vi "setColors.vi"(8 "error in (no error)":errorcluster, 10 "Colors":T1, 11 "Theme in":refnum<class "Theme.lvclass">) -> (0 "error out":errorcluster, 3 "Theme out":refnum<class "Theme.lvclass">)   [LabVIEW 2017, in "Theme.lvlib" / "Theme.lvclass"]
uses:
  Theme.lvclass
  Theme.Colors/Colors.ctl
  Theme.Colors/Theme.Colors.lvclass
  Theme.Colors/Theme.Colors.lvclass/Theme.Colors.ctl
  Theme.lvclass/Theme.ctl
  Theme.Colors/setContainer.vi
  Theme.Colors/setMain.vi
  Theme.Colors/setText.vi
  Theme.Font/Theme.Font.lvclass
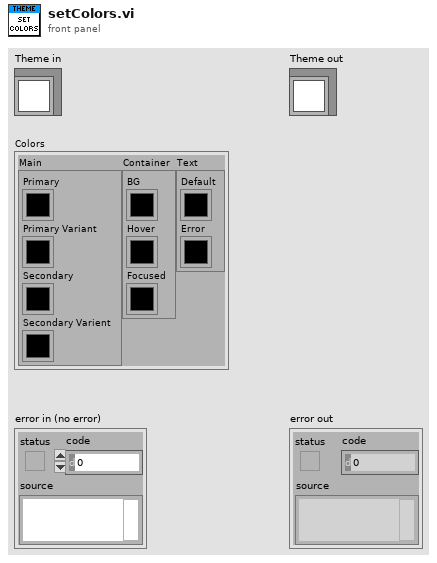
[diagram p1: front panel]
types:
  T1 = typedef "Theme.lvlib/Theme.Colors.lvclass/Colors.ctl" = cluster{"Main":cluster{"Primary":u32, "Primary Variant":u32, "Secondary":u32, "Secondary Varient":u32}, "Container":cluster{"BG":u32, "Hover":u32, "Focused":u32}, "Text":cluster{"Default":u32, "Error":u32}}
  T2 = typedef "Theme.lvlib/Theme.lvclass/Private Data.ctl" = cluster{"Colors":refnum<class "Theme.Colors.lvclass">, "Font":refnum<class "Theme.Font.lvclass">}
  T3 = cluster{"Primary":u32, "Primary Variant":u32, "Secondary":u32, "Secondary Varient":u32}
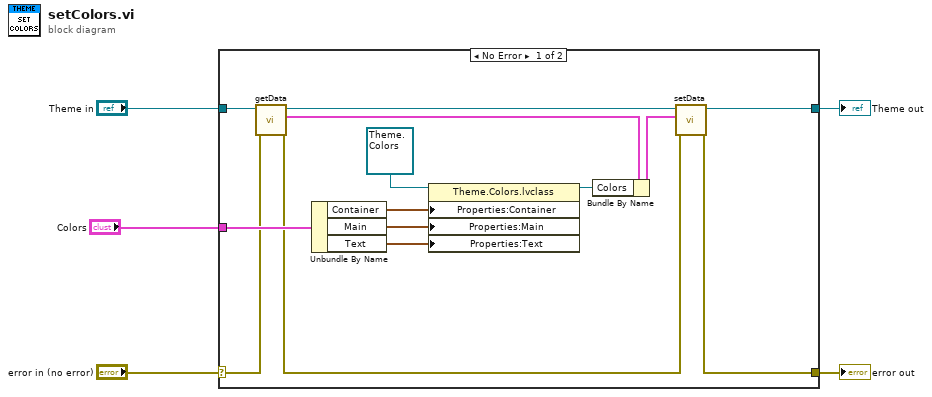
[diagram p0: block diagram]
diagram:
  n1 = case shown="No Error" "error in (no error)" {
    selector: "error in (no error)" -> [w8 w21]
    tunnel: [w6 w21] -> w4
    tunnel: [w18 w20] -> w2
    tunnel: "Theme in" -> [w17 w20]
    tunnel: "Colors" -> [w12 _]
    frame No Error {
      n2 = call "getData.vi"("error in (no error)"=w8, "Theme in"=w17) -> ("error out"=w7:errorcluster, "Theme"=w16:T2, "Theme out"=w19:refnum<class "Theme.lvclass">)  [unwired: 7 in]
      n3 = Unbundle By Name(w12) -> ("Container"=w11:cluster{"BG":u32, "Hover":u32, "Focused":u32}, "Main"=w10:T3, "Text"=w9:cluster{"Default":u32, "Error":u32})
      n4 = property class="Theme.Colors.lvclass"(reference=refnum<class "Theme.Colors.lvclass"> refnum ("Theme.lvlib:Theme.Colors.lvclass"), "Properties:Container"=w11, "Properties:Main"=w10, "Properties:Text"=w9) -> (reference out=w13:refnum<class "Theme.Colors.lvclass">)  [unwired: 1 in, 1 out]
      n5 = Bundle By Name(cluster=w16, "Colors"=w13) -> (w15:T2)
      n6 = call "setData.vi"("error in (no error)"=w7, "Theme"=w15, "Theme in"=w19) -> ("error out"=w6:errorcluster, "Theme out"=w18:refnum<class "Theme.lvclass">)  [unwired: 7 in]
    }
    frame Error {
    }
  }
  "error out" <- w4
  "Theme out" <- w2
